vi "Throw Error if Invalid Path.vi"(8 "error in":errorcluster, 10 "file path":path, 11 "File Ref in":T1 format="%.0x") -> (0 "error out":errorcluster, 3 "File Ref out":T1 format="%.0x")   [LabVIEW 2019, in "Telemetry System Explorer.lvlib"]
uses:
  Telemetry System Explorer.lvlib
  <vilib>/NI VeriStand/Custom Device API/Custom Device API.lvlib
  <vilib>/NI VeriStand/Custom Device API/Custom Device Item Ref.ctl
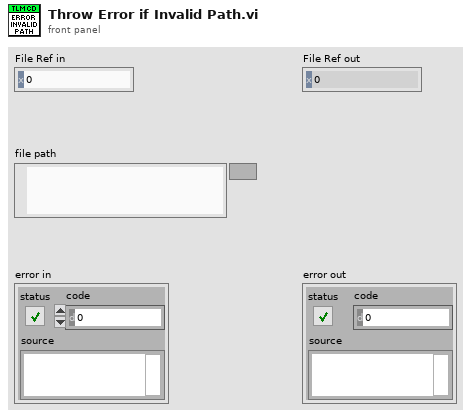
[diagram p1: front panel]
types:
  T1 = typedef "Custom Device API.lvlib/Custom Device Item Ref.ctl" = u64
  T2 = typedef "Custom Device API.lvlib/Custom Device Target Type.ctl" = enum16{"PharLap", "VxWorks", "Windows", "Linux_32_ARM", "Linux_x64"}
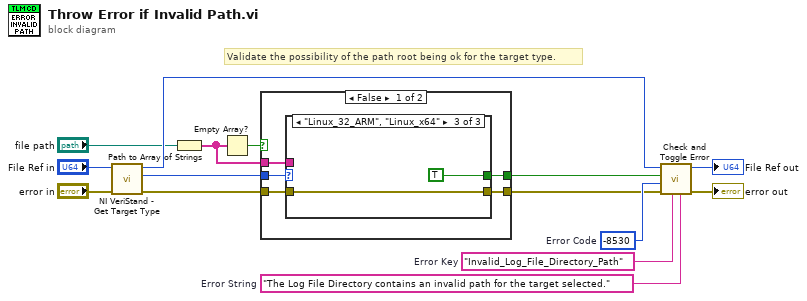
[diagram p0: block diagram]
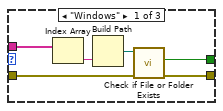
[diagram p2: hidden frame]
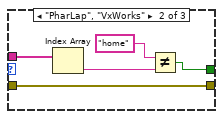
[diagram p3: hidden frame]
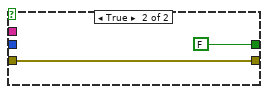
[diagram p4: hidden frame]
diagram:
  w13 = "The Log File Directory contains an invalid path for the target selected."  # Error String
  w14 = "Invalid_Log_File_Directory_Path"  # Error Key
  w15 = -8530  # Error Code
  # "Validate the possibility of the path root being ok for the target type."
  n1 = call <vilib>:"NI VeriStand - Get Target Type.vi"("error in (no error)"="error in", "Item Ref in"="File Ref in") -> ("error out"=w5:errorcluster, "Target Type"=w4:T2, "Item Ref out"=w10:T1)  [unwired: 7 in]
  n2 = Path to Array of Strings(0:"file path") -> (2:w9:string[])  [unwired: 1 out]
  n3 = Empty Array?(array=w9) -> (empty?=w8:bool)
  n4 = case shown="False" w8 {
    tunnel: w4 -> [w20 _]
    tunnel: [w19 FALSE ("file or folder exists?")] -> w7
    tunnel: w5 -> [w18 w35]
    tunnel: [w17 w35] -> w3
    tunnel: w9 -> [w16 _]
    frame False {
      n5 = case shown="\"Linux_32_ARM\", \"Linux_x64\"" w20 {
        tunnel: w16 -> [w26 w31 _]
        tunnel: [w24 w27 TRUE ("file or folder exists?")] -> w19
        tunnel: w18 -> [w23 w30 w32]
        tunnel: [w22 w30 w32] -> w17
        frame "Windows" {
          n6 = Index Array(array=w26) -> (element=w25:string)  [unwired: 1 in]
          n7 = Build Path(name or relative path=w25) -> (appended path=w21:path)  [unwired: 1 in]
          n8 = call <vilib>:"Check if File or Folder Exists.vi"("error in (no error)"=w23, "path"=w21) -> ("error out"=w22:errorcluster, "file or folder exists?"=w24:bool)  [unwired: 7 in, 1 out]
        }
        frame "PharLap", "VxWorks" {
          n9 = Index Array(array=w31) -> (element=w29:string)  [unwired: 1 in]
          n10 = Not Equal?(x="home", y=w29) -> (x != y?=w27:bool)
        }
        frame "Linux_32_ARM", "Linux_x64" {
        }
      }
    }
    frame True {
    }
  }
  n11 = call "Check and Toggle Error.vi"("error string"=w13, "error key"=w14, "error In"=w3, "error code"=w15, "clear error"=w7, "item reference in"=w10) -> ("error out"=→"error out":errorcluster, "item reference out"=→"File Ref out":T1)  [unwired: 4 in]
